vi "Add VI to Project.vi"(8 "error in":errorcluster, 10 "Add VI to this Project":string, 11 "Reference of newly created VI or CTL":refnum<vi>) -> (0 "error out":errorcluster)   [LabVIEW 2021]
doc: "This VI adds a VI to a project.\n\nThis VI assumes that the newly created VI has already been saved to disk (i.e. already exists on disk)."
panel:
  # "Development\ncontrols/indicators useful for development and testing, but which are not outputs of the VI"
  # "Input\nInputs to the VI"
  # "Output\nOutputs of the VI"
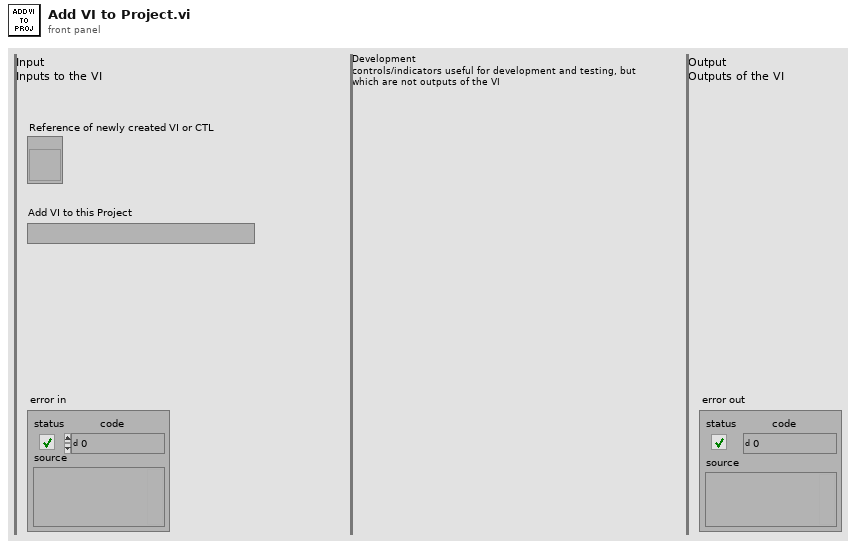
[diagram p1: front panel]
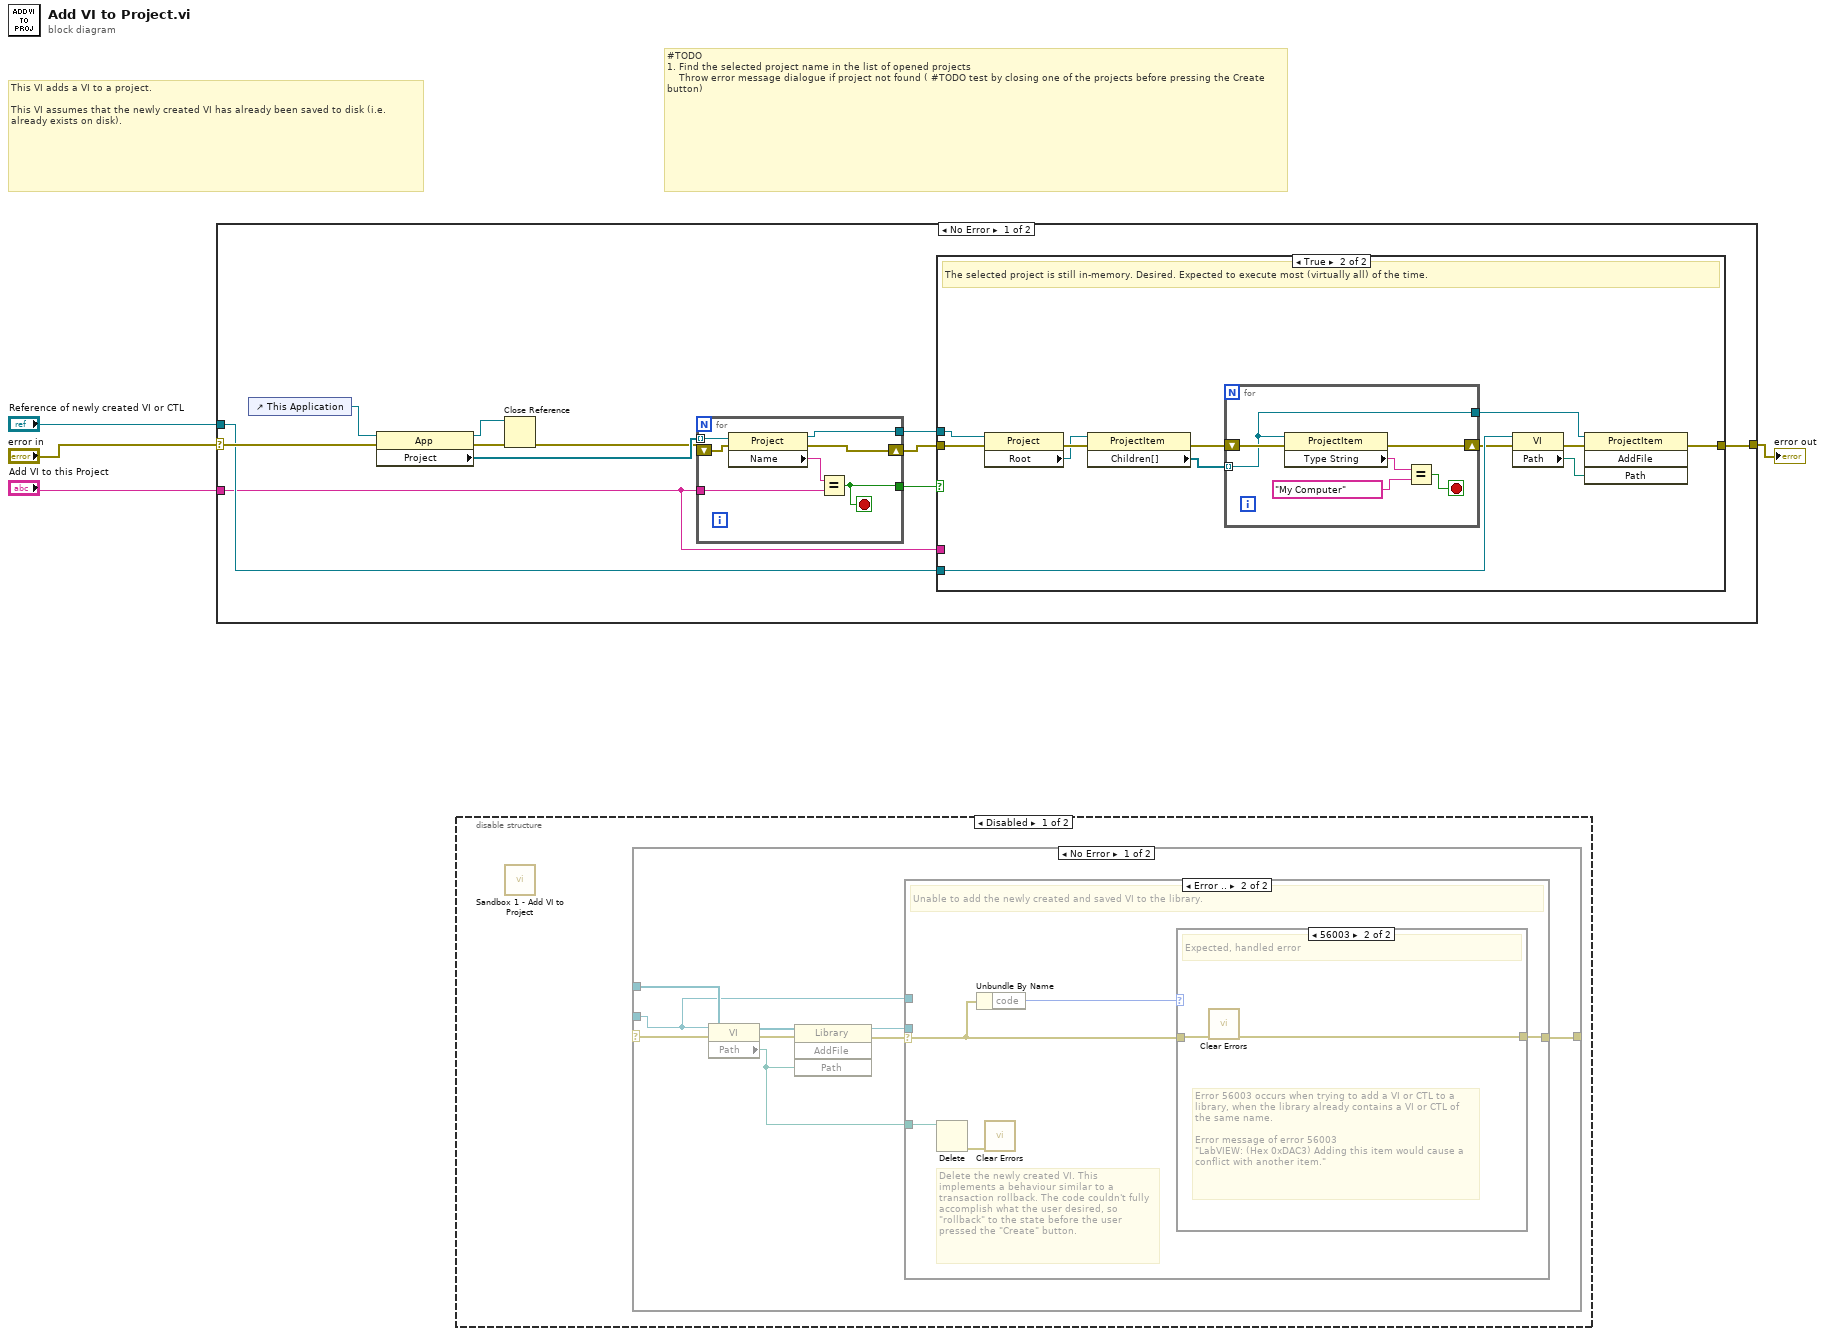
[diagram p0: block diagram]
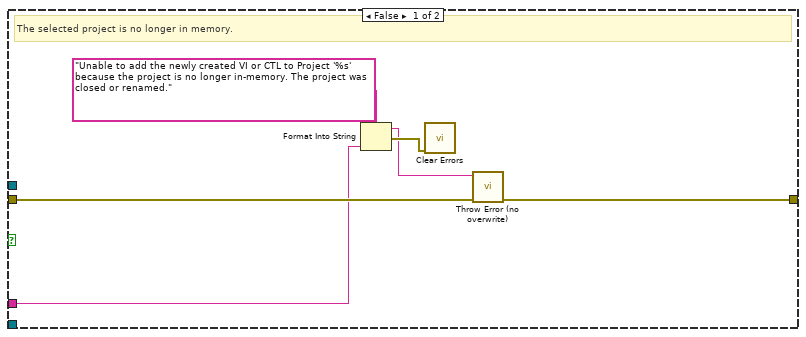
[diagram p2: hidden frame]
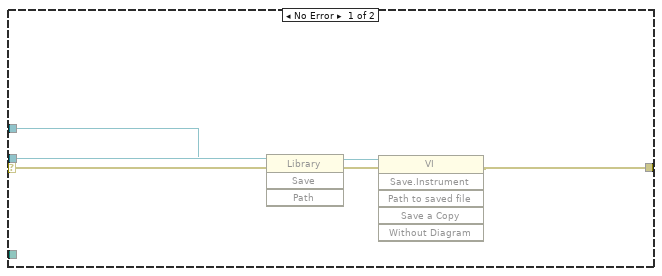
[diagram p4: hidden frame]
diagram:
  # "#TODO\n1. Find the selected project name in the list of opened projects\n    Throw error message dialogue if project not found ( #TODO test by closing one of the projects before pressing the Create button)"
  # "This VI adds a VI to a project.\n\nThis VI assumes that the newly created VI has already been saved to disk (i.e. already exists on disk)."
  n1 = case shown="No Error" "error in" {
    selector: "error in" -> [w15 w48]
    tunnel: [w16 w48] -> w3
    tunnel: "Reference of newly created VI or CTL" -> [w11 _]
    tunnel: "Add VI to this Project" -> [w5 _]
    frame No Error {
      n2 = control-ref of="This Application"() -> (w9:refnum<vi>)
      n3 = property class="App"(reference=w9, error in=w15) -> (reference out=w6:refnum<vi>, error out=w10:errorcluster, "Project"=w8:refnum<vi>[])
      n4 = Close Reference(reference=w6, error in (no error)=w10) -> (error out=w7:errorcluster)
      n5 = for {
        shift-right: [w22] -> w14
        shift-left: w7 -> [w23]
        tunnel: w8 -> [w21] mode=indexing
        tunnel: w5 -> [w19]
        tunnel: [w18] -> w13
        tunnel: [w17] -> w12
        stop <- w18 stop-if-true
        n6 = property class="Project"(reference=w21, error in=w23) -> (reference out=w17:refnum<vi>, error out=w22:errorcluster, "Name"=w20:string)
        n7 = Equal?(x=w20, y=w19) -> (x = y?=w18:bool)
      }
      n8 = case shown="True" w13 {
        tunnel: [w28 w38] -> w16
        tunnel: w14 -> [w29 w41]
        tunnel: w12 -> [_ w39]
        tunnel: w11 -> [_ w37]
        tunnel: w5 -> [w25 _]
        frame False {
          # "The selected project is no longer in memory."
          n9 = Format Into String(format string="Unable to add the newly created VI or CTL to Project '%s' because the project is no longer in-memory. The project was closed or renamed." ("message"), w25) -> (resulting string=w24:string, error out=w26:errorcluster)  [unwired: 2 in]
          n10 = call <vilib>:"Clear Errors.vi"("error in (no error)"=w26) -> ()  [unwired: 5 in, 2 out]
          n11 = call "Throw Error (no overwrite).vi"("error in"=w29, "Error Message"=w24) -> ("error out"=w28:errorcluster)  [unwired: 9 in]
        }
        frame True {
          # "The selected project is still in-memory. Desired. Expected to execute most (virtually all) of the time."
          n12 = property class="Project"(reference=w39, error in=w41) -> (error out=w40:errorcluster, "Root"=w35:refnum<vi>)  [unwired: 1 out]
          n13 = property class="ProjectItem"(reference=w35, error in=w40) -> (error out=w34:errorcluster, "Children[]"=w33:refnum<vi>[])  [unwired: 1 out]
          n14 = for {
            shift-right: [w46] -> w31
            shift-left: w34 -> [w47]
            tunnel: w33 -> [w42] mode=indexing
            tunnel: [w42] -> w32
            stop <- w43 stop-if-true
            n15 = property class="ProjectItem"(reference=w42, error in=w47) -> (error out=w46:errorcluster, "Type String"=w45:string)  [unwired: 1 out]
            n16 = Equal?(x=w45, y="My Computer") -> (x = y?=w43:bool)
          }
          n17 = property class="VI"(reference=w37, error in=w31) -> (error out=w30:errorcluster, "Path"=w36:path)  [unwired: 1 out]
          n18 = invoke class="ProjectItem" method="AddFile"(reference=w32, error in=w30, "Path"=w36) -> (error out=w38:errorcluster)  [unwired: 1 in, 3 out]
        }
      }
    }
    frame Error {
    }
  }
  "error out" <- w3
  n19 = disable-structure shown="Disabled" {
    frame Disabled {
      n20 = call "Sandbox 1 - Add VI to Project.vi"() -> ()  [unwired: 11 in, 1 out]
      n21 = case shown="No Error" {
        selector: _ -> [w54 w70]
        tunnel: [w53 w70] -> _
        tunnel: _ -> [w52 _]
        tunnel: _ -> [w50 _]
        frame No Error {
          n22 = property class="VI"(reference=w50, error in=w54) -> (error out=w51:errorcluster, "Path"=w49:path)  [unwired: 1 out]
          n23 = invoke class="Library" method="AddFile"(reference=w52, error in=w51, "Path"=w49) -> (reference out=w55:refnum<vi>, error out=w56:errorcluster)  [unwired: 1 in, 2 out]
          n24 = case shown="Error .." w56 {
            selector: w56 -> [w61 w64]
            tunnel: w55 -> [w59 _]
            tunnel: [w58 w65] -> w53
            tunnel: w50 -> [w57 _]
            tunnel: w49 -> [_ w63]
            frame No Error {
              n25 = invoke class="Library" method="Save"(reference=w59, error in=w61) -> (error out=w60:errorcluster)  [unwired: 2 in, 3 out]
              n26 = invoke class="VI" method="Save.Instrument"(reference=w57, error in=w60) -> (error out=w58:errorcluster)  [unwired: 4 in, 5 out]
            }
            frame Error {
              # "Delete the newly created VI. This implements a behaviour similar to a transaction rollback. The code couldn't fully accomplish what the user desired, so \"rollback\" to the state before the user pressed the \"Create\" button."
              # "Unable to add the newly created and saved VI to the library."
              n27 = Delete(path (use dialog)=w63) -> (error out=w62:errorcluster)  [unwired: 4 in, 2 out]
              n28 = Unbundle By Name(w64) -> ("code"=w66:i32)
              n29 = call <vilib>:"Clear Errors.vi"("error in (no error)"=w62) -> ()  [unwired: 5 in, 2 out]
              n30 = case shown="56003" w66 {
                tunnel: w64 -> [w67 w69]
                tunnel: [w67 w68] -> w65
                frame Default {
                  # "Do nothing. The error will be handled downstream."
                  # "Unexpected error"
                }
                frame 56003 {
                  # "Error 56003 occurs when trying to add a VI or CTL to a library, when the library already contains a VI or CTL of the same name.\n\nError message of error 56003\n\"LabVIEW: (Hex 0xDAC3) Adding this item would cause a conflict with another item.\""
                  # "Expected, handled error"
                  n31 = call <vilib>:"Clear Errors.vi"("error in (no error)"=w69) -> ("error out"=w68:errorcluster)  [unwired: 5 in, 1 out]
                }
              }
            }
          }
        }
        frame Error {
        }
      }
    }
    frame Enabled {
    }
  }
